vi "User Event LV2.vi"(0 "Stop":bool=TRUE, 11 "Error In":errorcluster, 13 "User event controls":T1) -> (4 "Stop Ref":refnum<user-event>, 6 "Run Ref":refnum<user-event>, 15 "Error Out":errorcluster)   [LabVIEW 2020, in "Test.lvclass"]
uses:
  Test.lvclass
  Typedef/User Event Controls.ctl
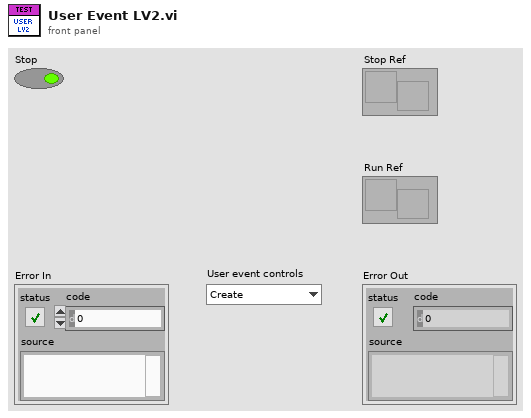
[diagram p1: front panel]
types:
  T1 = typedef "Test.lvclass/User Event Controls.ctl" = enum16{"Create", "Generate", "Run Test", "Get Ref", "Destroy"}
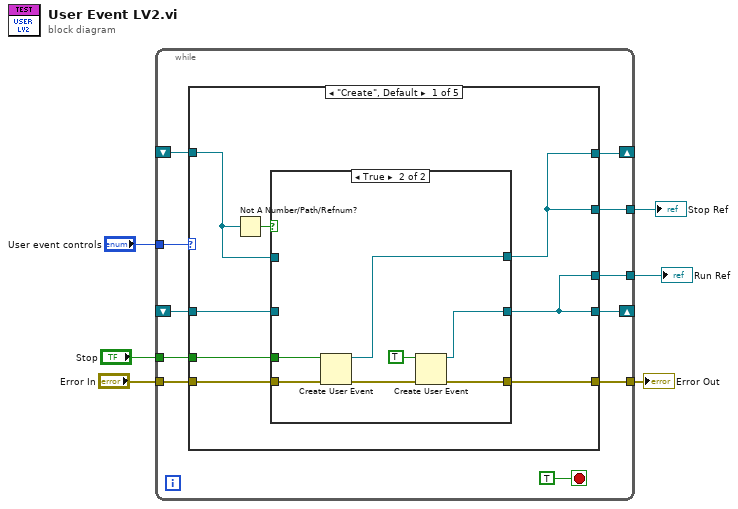
[diagram p0: block diagram]
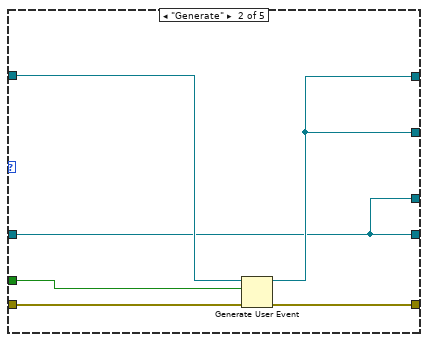
[diagram p3: hidden frame]
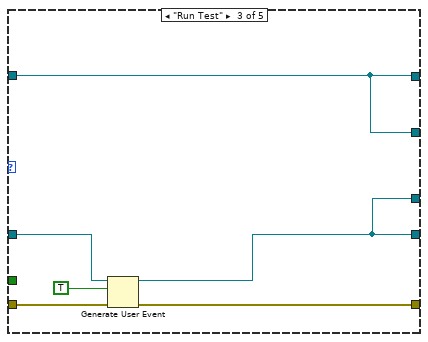
[diagram p4: hidden frame]
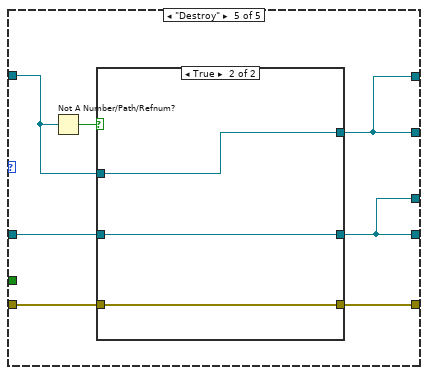
[diagram p6: hidden frame]
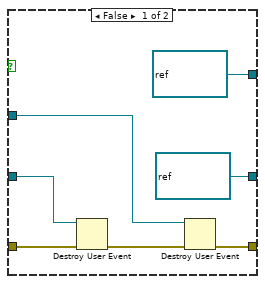
[diagram p7: hidden frame]
diagram:
  n1 = while {
    tunnel: "User event controls" -> [w17]
    tunnel: "Stop" -> [w15]
    shift-right: [w14] -> _
    shift-left: _ -> [w10]
    tunnel: "Error In" -> [w13]
    tunnel: [w12] -> w4
    tunnel: [w11] -> w3
    shift-right: [w9] -> _
    shift-left: _ -> [w8]
    tunnel: [w7] -> w2
    stop <- TRUE stop-if-true
    n2 = case shown="\"Create\", Default" w17 {
      tunnel: w15 -> [w25 w39 _ _ _]
      tunnel: [w20 w38 w44 w50 w53] -> w14
      tunnel: w10 -> [w23 w40 w44 w50 w56]
      tunnel: w13 -> [w22 w37 w47 w49 w57]
      tunnel: [w21 w41 w46 w49 w54] -> w12
      tunnel: [w20 w38 w44 w50 w53] -> w11
      tunnel: [w18 w36 w42 w48 w51] -> w9
      tunnel: w8 -> [w19 w36 w45 w48 w52]
      tunnel: [w18 w36 w42 w48 w51] -> w7
      frame "Create", Default {
        n3 = Not A Number/Path/Refnum?(number/path/refnum=w23) -> (NaN/Path/Refnum?=w24:bool)
        n4 = case shown="True" w24 {
          tunnel: w25 -> [_ w35]
          tunnel: [w28 w33] -> w20
          tunnel: w23 -> [w28 _]
          tunnel: w22 -> [w27 w34]
          tunnel: [w27 w31] -> w21
          tunnel: [w26 w29] -> w18
          tunnel: w19 -> [w26 _]
          frame False {
          }
          frame True {
            n5 = Create User Event(user event datatype=w35, error in=w34) -> (user event=w33:refnum<user-event>, error out=w32:errorcluster)
            n6 = Create User Event(user event datatype=TRUE ("Run Test?"), error in=w32) -> (user event=w29:refnum<user-event>, error out=w31:errorcluster)
          }
        }
      }
      frame "Generate" {
        n7 = Generate User Event(user event=w40, event data cluster=w39, error in=w37) -> (user event out=w38:refnum<user-event>, error out=w41:errorcluster)  [unwired: 1 in]
      }
      frame "Run Test" {
        n8 = Generate User Event(user event=w45, event data cluster=TRUE ("event data"), error in=w47) -> (user event out=w42:refnum<user-event>, error out=w46:errorcluster)  [unwired: 1 in]
      }
      frame "Get Ref" {
      }
      frame "Destroy" {
        n9 = Not A Number/Path/Refnum?(number/path/refnum=w56) -> (NaN/Path/Refnum?=w55:bool)
        n10 = case shown="True" w55 {
          tunnel: w57 -> [w61 w67]
          tunnel: w56 -> [w64 w66]
          tunnel: [w63 w67] -> w54
          tunnel: [refnum<user-event> refnum ("Stop") w66] -> w53
          tunnel: w52 -> [w59 w65]
          tunnel: [refnum<user-event> refnum ("Run Test?") w65] -> w51
          frame False {
            n11 = Destroy User Event(user event=w59, error in=w61) -> (error out=w60:errorcluster)
            n12 = Destroy User Event(user event=w64, error in=w60) -> (error out=w63:errorcluster)
          }
          frame True {
          }
        }
      }
    }
  }
  "Error Out" <- w4
  "Stop Ref" <- w3
  "Run Ref" <- w2
